vi "KundtsTubeJ&J.vi"() -> ()   [LabVIEW 2015]
panel:
  out "Waveform Graph":dbl[](graph)
  in  "Sampling Rate":dbl
  in  "#of Samples":dbl
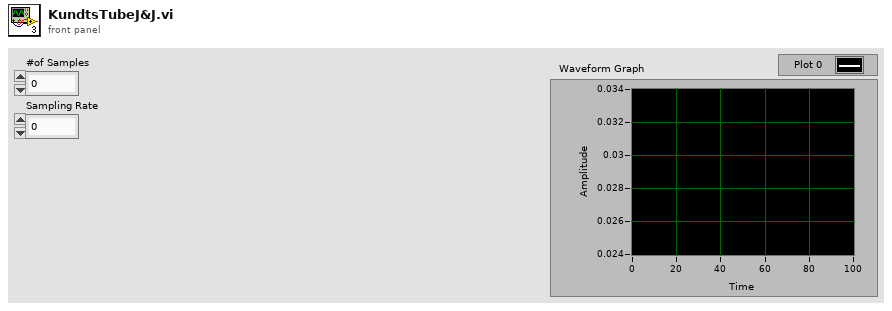
[diagram p1: front panel]
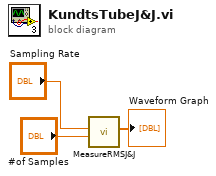
[diagram p0: block diagram]
diagram:
  n1 = call "MeasureRMSJ&J.vi"("#of Samples"="#of Samples", "Sampling Rate"="Sampling Rate") -> ("Waveform Graph"=→"Waveform Graph":dbl[])  [unwired: 9 in]
